vi "save_xml.vi"(7 "base path":path, 8 "error in":errorcluster, 9 "Array of DDS Boxes":T1, 11 "Enable DDS":bool=TRUE) -> (0 "error out":errorcluster)   [LabVIEW 2012, in "DDS.lvclass"]
uses:
  DDS.lvclass
  DDS drivers v3/Array_of_DDS_Boxes.ctl
  DDS drivers v3/DDS_box_cluster.ctl
  DDS drivers v3/DDS_box_device_reference.ctl
  <vilib>/ni845x/ni845x.llb/ni845xControl.ctl
  DDS drivers v3/DDS RAM mode.ctl
  <vilib>/Utility/xml.llb/Write to XML File(string).vi
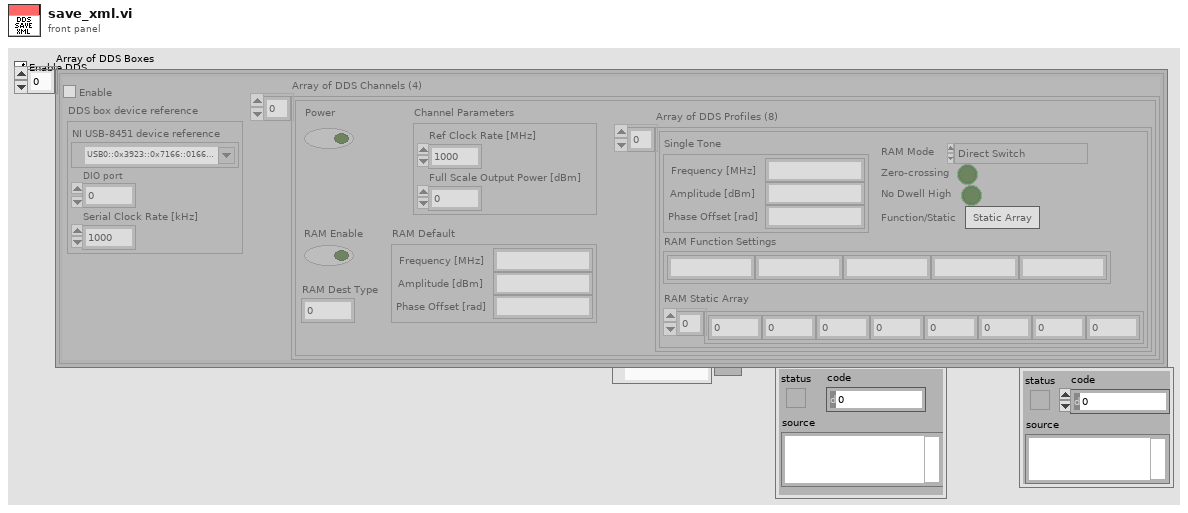
[diagram p1: front panel]
types:
  T1 = typedef "Array_of_DDS_Boxes.ctl" = T2[]
  T2 = typedef "DDS_box_cluster.ctl" = cluster{"DDS box device reference":T3, "Array of DDS Channels (4)":cluster{"Power":bool, "Channel Parameters":cluster{"Ref Clock Rate [MHz]":dbl, "Full Scale Output Power [dBm]":dbl}, "RAM Enable":bool, "RAM Dest Type":u8, "RAM Default":cluster{"Frequency [MHz]":string, "Amplitude [dBm]":string, "Phase Offset [rad]":string}, "Array of DDS Profiles (8)":cluster{"Single Tone":cluster{"Frequency [MHz]":string, "Amplitude [dBm]":string, "Phase Offset [rad]":string}, "RAM Mode ":T5, "Zero-crossing":bool, "No Dwell High":bool, "Function/Static":bool, "RAM Function Settings":string[], "RAM Static Array":dbl[]}[]}[], "Enable":bool}
  T3 = typedef "DDS_box_device_reference.ctl" = cluster{"NI USB-8451 device reference":T4, "DIO port":u8, "Serial Clock Rate [kHz]":u16}
  T4 = typedef "ni845xControl.ctl" = refnum<k21>
  T5 = typedef "DDS RAM mode.ctl" = enum16{"Direct Switch", "Ramp Up", "Bidirectional Ramp", "Continuous Bidirectional Ramp", "Continuous Recirculate", "Direct Switch 2", "Direct Switch 3", "Direct Switch 4"}
  T6 = cluster{"Enable DDS":bool, "Array of DDS Boxes":T1}
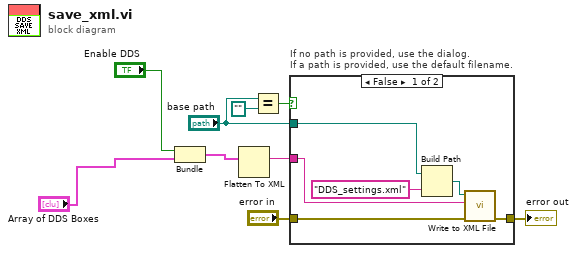
[diagram p0: block diagram]
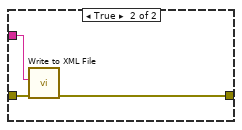
[diagram p2: hidden frame]
diagram:
  n1 = Bundle("Enable DDS"="Enable DDS", "Array of DDS Boxes"="Array of DDS Boxes") -> (w2:T6)  [unwired: 1 in]
  n2 = Flatten To XML(anything=w2) -> (xml string=w4:string)
  n3 = Equal?(x="base path", y=path "") -> (x = y?=w7:bool)
  n4 = case "If no path is provided, use the dialog.\nIf a path is provided, use the default filename." shown="False" w7 {
    tunnel: [w11 w17] -> w8
    tunnel: "base path" -> [w14 _]
    tunnel: "error in" -> [w12 w18]
    tunnel: w4 -> [w10 w16]
    frame False {
      n5 = Build Path(base path=w14, name or relative path="DDS_settings.xml") -> (appended path=w13:path)
      n6 = call-poly <vilib>:"Write to XML File.vi"("error in (no error)"=w12, "XML Input"=w10, "XML File Path"=w13) -> ("error out"=w11:errorcluster)  [unwired: 6 in, 2 out]
    }
    frame True {
      n7 = call-poly <vilib>:"Write to XML File.vi"("error in (no error)"=w18, "XML Input"=w16) -> ("error out"=w17:errorcluster)  [unwired: 7 in, 2 out]
    }
  }
  "error out" <- w8
